vi "Reserve Sessions - 1Pin.vi"(6 "timeout (ms)":i32, 8 "error in":errorcluster, 10 "pin or relay name":string, 11 "measurement context in":refnum<class "Measure Call Context.lvclass">) -> (0 "error out":errorcluster, 2 "session reservation out":refnum<class "Session Reservation.lvclass">, 3 "measurement context out":refnum<class "Measure Call Context.lvclass">)   [LabVIEW 2021, in "NI Measurement Plug-In SDK.lvlib" / "Measure Call Context.lvclass"]
doc: "Reserves session(s) based on the provided pin information."
uses:
  Measure Call Context.lvclass
  Clients/Session Management V1/Session Reservation/Session Reservation.lvclass
  Helpers/Error Strings Global Internal.vi
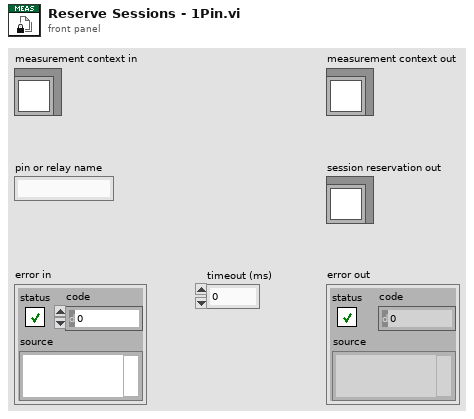
[diagram p1: front panel]
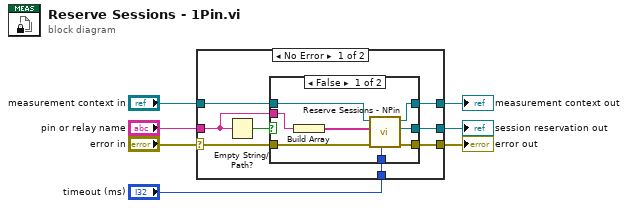
[diagram p0: block diagram]
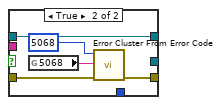
[diagram p2: hidden frame]
diagram:
  n1 = case shown="No Error" "error in" {
    selector: "error in" -> [w13 w30]
    tunnel: [w11 w30] -> w6
    tunnel: [w14 w29] -> w4
    tunnel: "measurement context in" -> [w15 w29]
    tunnel: "pin or relay name" -> [w8 _]
    tunnel: "timeout (ms)" -> [w10 _]
    tunnel: [w12 _] -> w1
    frame No Error {
      n2 = Empty String/Path?(string/path=w8) -> (empty?=w9:bool)
      n3 = case shown="False" w9 {
        tunnel: w15 -> [w23 w24]
        tunnel: [w22 w24] -> w14
        tunnel: w13 -> [w21 w27]
        tunnel: [w19 _] -> w12
        tunnel: [w18 w28] -> w11
        tunnel: w10 -> [w17 _]
        tunnel: w8 -> [w16 _]
        frame False {
          n4 = Build Array(w16) -> (w20:string[])
          n5 = call "Reserve Sessions - NPin.vi"("timeout (ms)"=w17, "error in"=w21, "pin or relay names"=w20, "measurement context in"=w23) -> ("error out"=w18:errorcluster, "session reservation out"=w19:refnum<class "Session Reservation.lvclass">, "measurement context out"=w22:refnum<class "Measure Call Context.lvclass">)  [unwired: 5 in]
        }
        frame True {
          n6 = global read "Error Strings Global Internal.vi" "5068"() -> (w25:string)
          n7 = call <vilib>:"Error Cluster From Error Code.vi"("error in (no error)"=w27, "error message (\"\")"=w25, "error code (0)"=5068) -> ("error out"=w28:errorcluster)  [unwired: 6 in]
        }
      }
    }
    frame Error {
    }
  }
  "error out" <- w6
  "measurement context out" <- w4
  "session reservation out" <- w1
